vi "Ports Consructor.vi"(8 "error in (no error)":errorcluster, 9 "PortNames":string[](array[string]), 10 "Max port size":i32, 11 "Ports in":refnum<class "Ports.lvclass">) -> (0 "error out":errorcluster, 3 "Ports out":refnum<class "Ports.lvclass">)   [LabVIEW 2019, in "Ports.lvclass"]
uses:
  Ports.lvclass
  Ports.lvclass/Ports.ctl
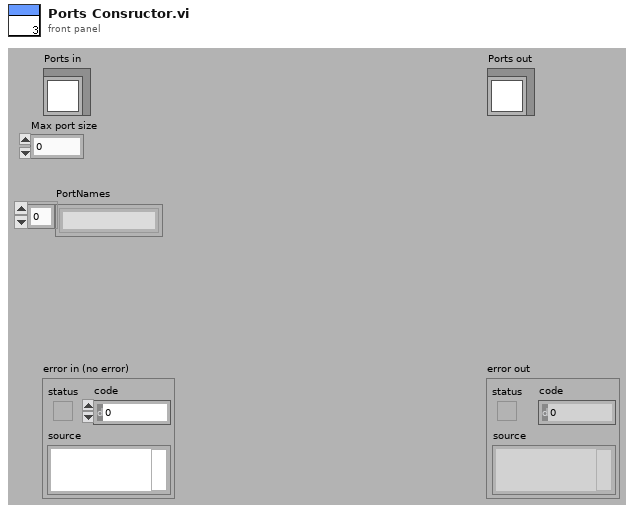
[diagram p1: front panel]
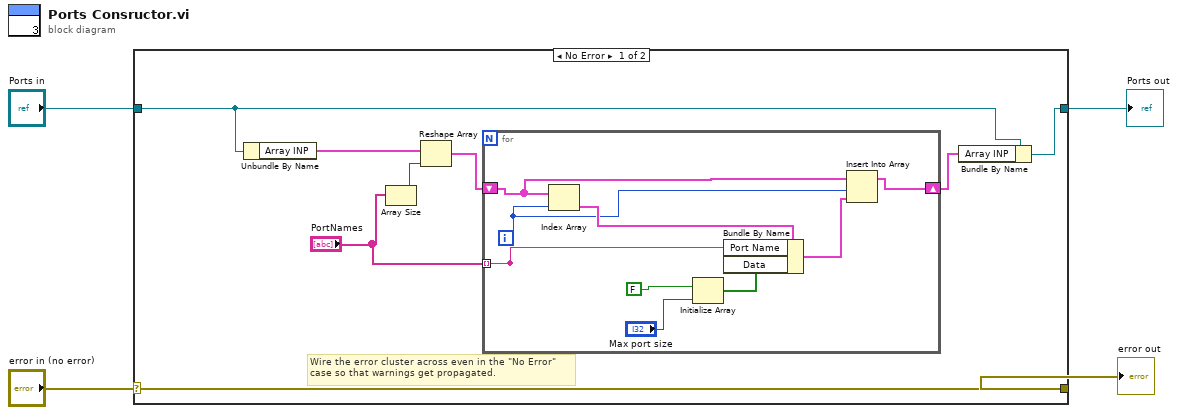
[diagram p0: block diagram]
diagram:
  n1 = case shown="No Error" "error in (no error)" {
    selector: "error in (no error)" -> [w12 w23]
    tunnel: [w12 w23] -> w3
    tunnel: [w5 w22] -> w1
    tunnel: "Ports in" -> [w7 w22]
    frame No Error {
      # "Wire the error cluster across even in the \"No Error\"\ncase so that warnings get propagated."
      n2 = Unbundle By Name(w7) -> ("Array INP"=w11:cluster{"Port Name":string, "Data":bool[]}[])
      n3 = Array Size(array="PortNames") -> (size(s)=w8:i32)
      n4 = Reshape Array(w11, w8) -> (w10:cluster{"Port Name":string, "Data":bool[]}[])
      n5 = for {
        tunnel: [w20] -> _ mode=indexing
        tunnel: "PortNames" -> [w20] mode=indexing
        shift-right: [w15] -> w6
        shift-left: w10 -> [w16]
        i -> [w13]
        n6 = Index Array(array=w16, index=w13) -> (element=w21:cluster{"Port Name":string, "Data":bool[]})
        n7 = Initialize Array(FALSE ("Boolean"), "Max port size") -> (w17:bool[])
        n8 = Bundle By Name(cluster=w21, "Port Name"=w20, "Data"=w17) -> (w14:cluster{"Port Name":string, "Data":bool[]})
        n9 = Insert Into Array(array=w16, index=w13, new element=w14) -> (w15:cluster{"Port Name":string, "Data":bool[]}[])
      }
      n10 = Bundle By Name(cluster=w7, "Array INP"=w6) -> (w5:refnum<class "Ports.lvclass">)
    }
    frame Error {
    }
  }
  "error out" <- w3
  "Ports out" <- w1
